vi "lumencor_on.vi"   [LabVIEW 2011]
uses:
  <vilib>/DAQmx/write.llb/DAQmx Write.vi
  <vilib>/DAQmx/write.llb/DAQmx Write (Analog 1D DBL NChan 1Samp).vi
  <vilib>/DAQmx/miscellaneous.llb/DAQmx Fill In Error Info.vi
types:
  T1 = enum32{"Invalid", "Standard", "Closed", "Hidden", "Minimized", "Maximized"}
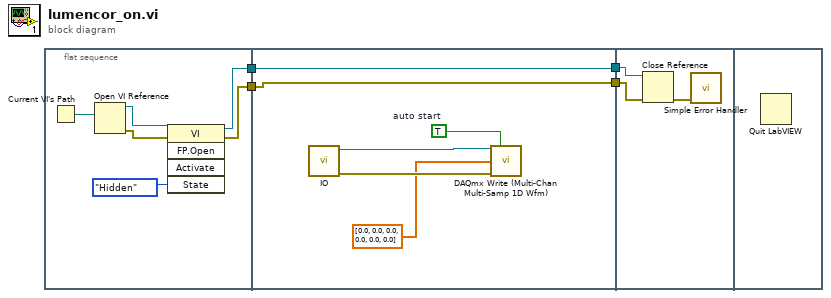
[diagram p0: block diagram]
diagram:
  n1 = flat-sequence {
    tunnel: [w6] -> w3
    tunnel: [w5] -> w2
    tunnel: [w12] -> w4
    tunnel: w3 -> [w12]
    tunnel: w2 -> [w11]
    tunnel: [w11] -> w1
    tunnel: w4 -> [w19]
    tunnel: w1 -> [w18]
    frame #0 {
      n2 = Current VI's Path() -> (path=w7:path)
      n3 = Open VI Reference(vi path=w7) -> (vi reference=w8:refnum<vi>, error out=w9:errorcluster)  [unwired: 5 in]
      n4 = invoke class="VI" method="FP.Open"(reference=w8, error in=w9, "State"=T1."Hidden") -> (reference out=w6:refnum<vi>, error out=w5:errorcluster)  [unwired: 2 in, 3 out]
    }
    frame #1 {
      w16 = TRUE  # auto start
      n5 = call "IO.vi"() -> ("error out"=w14:errorcluster, "task out"=w15:refnum<k21>)  [unwired: 10 in]
      n6 = call-poly "DAQmx Write (Multi-Chan Multi-Samp 1D Wfm).vi"("task/channels in"=w15, "auto start"=w16, "data"=dbl[] [0.0, 0.0, 0.0, 0.0, 0.0, 0.0], "error in"=w14) -> ()  [unwired: 12 out]
    }
    frame #2 {
      n7 = Close Reference(reference=w19, error in (no error)=w18) -> (error out=w17:errorcluster)
      n8 = call <vilib>:"Simple Error Handler.vi"("error in (no error)"=w17) -> ()  [unwired: 4 in, 5 out]
    }
    frame #3 {
      n9 = Quit LabVIEW() -> ()  [unwired: 1 in]
    }
  }
